vi "Delete Files from ZIP.vi"(7 "Temp Folder":path, 8 "error in":errorcluster, 10 "Files to Remove":string[](array[string]), 11 "Zip File Path":path) -> (0 "error out":errorcluster, 3 "Zip File Path Out":path)   [LabVIEW 2020]
uses:
  <vilib>/zip/NI_Unzip.lvlib
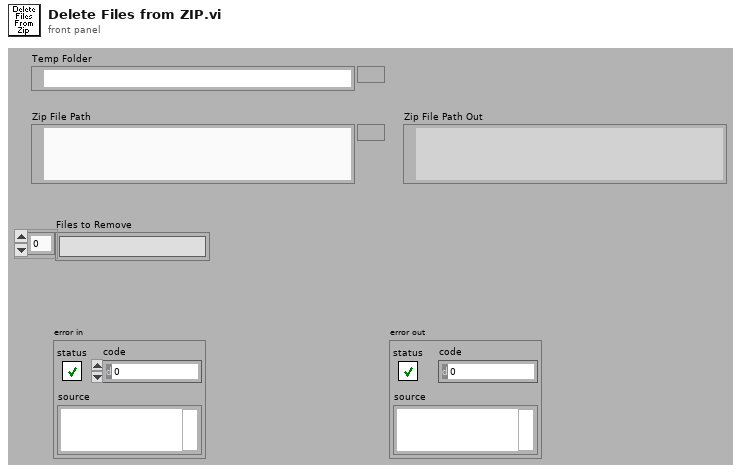
[diagram p1: front panel]
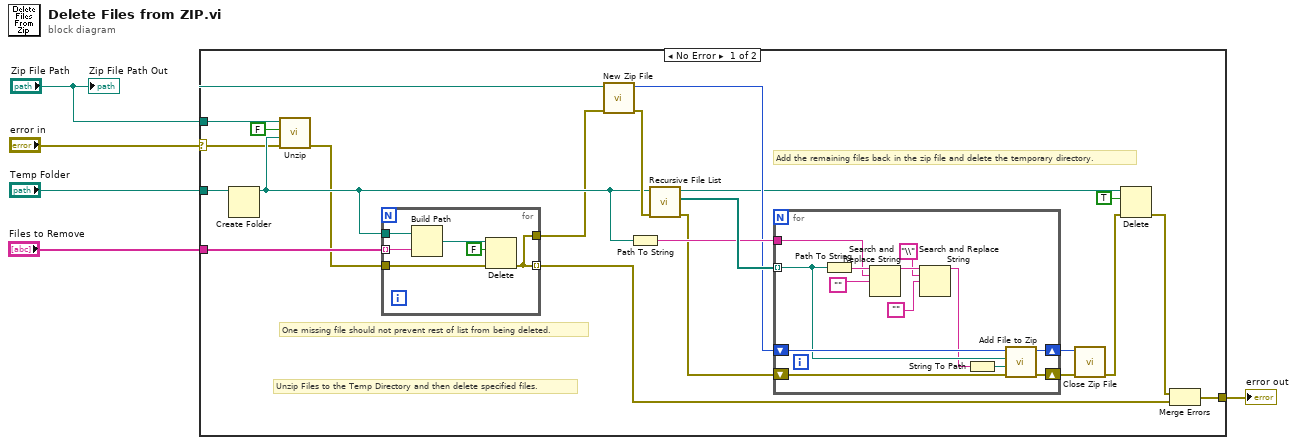
[diagram p0: block diagram]
diagram:
  n1 = case shown="No Error" "error in" {
    selector: "error in" -> [w6 w46]
    tunnel: "Temp Folder" -> [w14 _]
    tunnel: "Files to Remove" -> [w13 _]
    tunnel: "Zip File Path" -> [w12 _]
    tunnel: [w7 w46] -> w2
    frame No Error {
      # "One missing file should not prevent rest of list from being deleted."
      # "Add the remaining files back in the zip file and delete the temporary directory."
      # "Unzip Files to the Temp Directory and then delete specified files."
      n2 = Create Folder(path (use dialog)=w14) -> (created path=w15:path)  [unwired: 2 in, 2 out]
      n3 = call <vilib>:"Unzip.vi"("error in (no error)"=w6, "Target directory (same as Zip file if empty)"=w15, "Preview only?"=FALSE, "Zip file"=w12) -> ("error out"=w11:errorcluster)  [unwired: 5 in, 2 out]
      n4 = for {
        tunnel: w15 -> [w32]
        tunnel: w13 -> [w29] mode=indexing
        tunnel: w11 -> [w28]
        tunnel: [w27] -> w10 mode=indexing
        tunnel: [w27] -> w9
        n5 = Build Path(base path=w32, name or relative path=w29) -> (appended path=w31:path)
        n6 = Delete(path (use dialog)=w31, entire hierarchy (F)=FALSE, error in=w28) -> (error out=w27:errorcluster)  [unwired: 2 in, 2 out]
      }
      n7 = call <vilib>:"New Zip File.vi"("error in (no error)"=w9, "target"=w12) -> ("error out"=w22:errorcluster, "zip file out"=w23:i64)  [unwired: 3 in, 1 out]
      n8 = Path To String(path=w15) -> (string=w24:string)
      n9 = call <vilib>:"Recursive File List.vi"("error in (no error)"=w22, "Folder Path"=w15) -> ("error out"=w16:errorcluster, "All Files in Dir"=w25:path[], "dup Folder Path"=w21:path)  [unwired: 5 in, 2 out]
      n10 = for {
        tunnel: w25 -> [w38] mode=indexing
        tunnel: w24 -> [w40]
        shift-right: [w34] -> w20
        shift-left: w16 -> [w35]
        shift-right: [w33] -> w18
        shift-left: w23 -> [w39]
        n11 = Path To String(path=w38) -> (string=w44:string)
        n12 = Search and Replace String(input string=w44, search string=w40, replace string="") -> (result string=w42:string)  [unwired: 1 in, 7 out]
        n13 = Search and Replace String(input string=w42, search string="\\", replace string="") -> (result string=w37:string)  [unwired: 1 in, 7 out]
        n14 = String To Path(string=w37) -> (path=w36:path)
        n15 = call <vilib>:"Add File to Zip.vi"("error in (no error)"=w35, "destination path in zip"=w36, "source file path"=w38, "zip file in"=w39) -> ("error out"=w34:errorcluster, "zip file out"=w33:i64)  [unwired: 6 in]
      }
      n16 = call <vilib>:"Close Zip File.vi"("error in (no error)"=w20, "zip file in"=w18) -> ("error out"=w19:errorcluster)  [unwired: 5 in]
      n17 = Delete(path (use dialog)=w21, entire hierarchy (F)=TRUE, error in=w19) -> (error out=w8:errorcluster)  [unwired: 2 in, 2 out]
      n18 = Merge Errors(w8, w10) -> (w7:errorcluster)
    }
    frame Error {
    }
  }
  "error out" <- w2
  "Zip File Path Out" <- "Zip File Path"
